vi "initialise.vi"(8 "error in (no error)":errorcluster, 11 "GenericTrajectory in":refnum<class "TrajectoryDL110413StraightLine.lvclass">) -> (0 "error out":errorcluster, 3 "GenericTrajectory out":refnum<class "TrajectoryDL110413StraightLine.lvclass">)   [LabVIEW 2010, in "TrajectoryDL110413StraightLine.lvclass"]
uses:
  TrajectoryDL110413StraightLine.lvclass
  TrajectoryDL091126GenericVoxel/TrajectoryDL091126GenericVoxel/TrajectoryDL091126GenericVoxel.lvclass
  common/enumerations/x_y_z_enumeration.ctl
  common/enumerations/functional_global_action_enum.ctl
  TrajectoryDL110413StraightLine.lvclass/TrajectoryDL110413StraightLine.ctl
  common/classes/ImageCollection/ImageCollection/ImageCollection.lvclass
  common/classes/Image/Image/Image.lvclass
  <vilib>/Analysis/1siggen.llb/Ramp Pattern by Samples.vi
  <vilib>/Analysis/NI_AALBase.lvlib
  common/classes/SpaceVector/SpaceVector/SpaceVector.lvclass
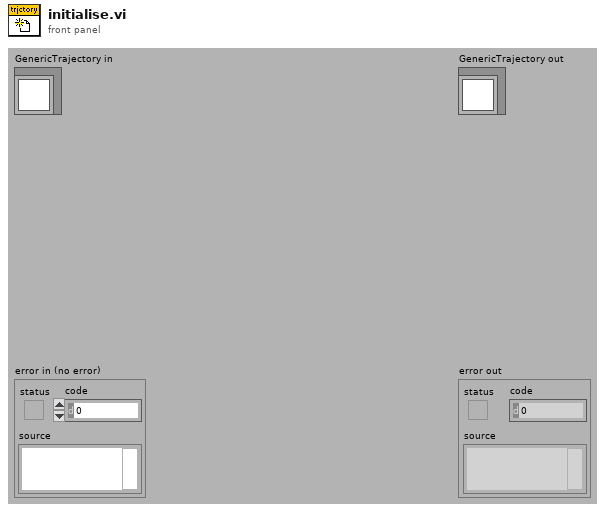
[diagram p1: front panel]
types:
  T1 = typedef "x_y_z_enumeration.ctl" = enum16{"x", "y", "z"}
  T2 = typedef "functional_global_action_enum.ctl" = enum16{"get", "set", "reset"}
  T3 = cluster{"guide points[0]":refnum<class "SpaceVector.lvclass">, "guide points[1]":refnum<class "SpaceVector.lvclass">}
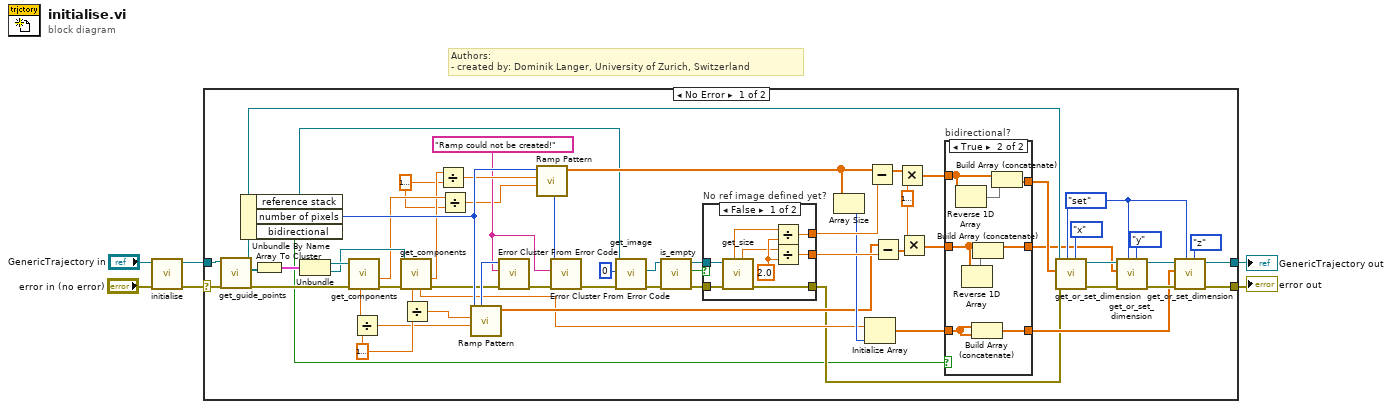
[diagram p0: block diagram]
diagram:
  # "Authors: \n- created by: Dominik Langer, University of Zurich, Switzerland"
  n1 = call-parent "initialise.vi"("error in (no error)"="error in (no error)", "GenericTrajectory in"="GenericTrajectory in") -> ("error out"=w4:errorcluster, "GenericTrajectory out"=w3:refnum<class "TrajectoryDL110413StraightLine.lvclass">)  [unwired: 8 in]
  n2 = case shown="No Error" w4 {
    selector: w4 -> [w47 w87]
    tunnel: w3 -> [w46 w88]
    tunnel: [w60 w88] -> w2
    tunnel: [w58 w87] -> w1
    frame No Error {
      w25 = dbl[unit] 1e-06 ("y")
      w19 = "Ramp could not be created!" ("error message (\"\")")
      w15 = dbl[unit] 1e-06 ("y")
      w28 = dbl[unit] 1e-06 ("y")
      w57 = functional_global_action_enum."set" ("action")
      n3 = call-dynamic "get_guide_points.vi"("error in (no error)"=w47, "TrajectoryDL110413StraightLine in"=w46) -> ("error out"=w33:errorcluster, "guide points"=w44:refnum<class "SpaceVector.lvclass">[], "TrajectoryDL110413StraightLine out"=w45:refnum<class "TrajectoryDL110413StraightLine.lvclass">)  [unwired: 7 in]
      n4 = Unbundle By Name(w45) -> ("reference stack"=w18:refnum<class "ImageCollection.lvclass">, "number of pixels"=w66:i32, "bidirectional"=w7:bool)
      n5 = Array To Cluster(array=w44) -> (cluster=w43:T3)
      n6 = Unbundle(w43) -> ("guide points[0]"=w35:refnum<class "SpaceVector.lvclass">, "guide points[1]"=w34:refnum<class "SpaceVector.lvclass">)
      n7 = call "get_components.vi"("error in (no error)"=w33, "SpaceVector in"=w35) -> ("error out"=w30:errorcluster, "x"=w27:dbl[unit], "y"=w31:dbl[unit])  [unwired: 4 in, 3 out]
      n8 = Divide(x=w31, y=w28) -> (x/y=w23:dbl)
      n9 = call "get_components.vi"("error in (no error)"=w30, "SpaceVector in"=w34) -> ("error out"=w21:errorcluster, "x"=w26:dbl[unit], "z"=w32:dbl[unit], "y"=w29:dbl[unit])  [unwired: 4 in, 2 out]
      n10 = Divide(x=w29, y=w28) -> (x/y=w22:dbl)
      n11 = Divide(x=w26, y=w25) -> (x/y=w24:dbl)
      n12 = Divide(x=w27, y=w25) -> (x/y=w17:dbl)
      n13 = call-poly <vilib>:"Ramp Pattern.vi"("start"=w23, "end"=w22, "samples"=w66) -> ("error"=w42:i32, "Ramp Pattern"=w36:dbl[])  [unwired: 7 in]
      n14 = call <vilib>:"Error Cluster From Error Code.vi"("error in (no error)"=w21, "error message (\"\")"=w19, "error code (0)"=w42) -> ("error out"=w40:errorcluster)  [unwired: 6 in]
      n15 = call-poly <vilib>:"Ramp Pattern.vi"("start"=w17, "end"=w24, "samples"=w66) -> ("error"=w41:i32, "Ramp Pattern"=w38:dbl[])  [unwired: 7 in]
      n16 = call <vilib>:"Error Cluster From Error Code.vi"("error in (no error)"=w40, "error message (\"\")"=w19, "error code (0)"=w41) -> ("error out"=w20:errorcluster)  [unwired: 6 in]
      n17 = call-dynamic "get_image.vi"("error in (no error)"=w20, "index"=0, "ImageCollection in"=w18) -> ("error out"=w52:errorcluster, "Image.lvclass"=w50:refnum<class "Image.lvclass">)  [unwired: 6 in, 1 out]
      n18 = call-dynamic "is_empty.vi"("error in (no error)"=w52, "Image in"=w50) -> ("error out"=w51:errorcluster, "emtpy?"=w48:bool, "Image out"=w49:refnum<class "Image.lvclass">)  [unwired: 7 in]
      n19 = case "No ref image defined yet?" shown="False" w48 {
        tunnel: [w85 w86] -> w8
        tunnel: [w82 _] -> w54
        tunnel: [w80 _] -> w53
        tunnel: w51 -> [w79 w86]
        tunnel: w49 -> [w78 _]
        frame False {
          w84 = 2.0 ("y")
          n20 = call-dynamic "get_size.vi"("error in (no error)"=w79, "Image in"=w78) -> ("error out"=w85:errorcluster, "physical size y"=w81:dbl, "physical size x"=w83:dbl)  [unwired: 2 in, 5 out]
          n21 = Divide(x=w83, y=w84) -> (x/y=w82:dbl)
          n22 = Divide(x=w81, y=w84) -> (x/y=w80:dbl)
        }
        frame True {
        }
      }
      n23 = Array Size(array=w38) -> (size(s)=w39:i32)
      n24 = Initialize Array(w32, w39) -> (w12:dbl[unit][])
      n25 = Subtract(x=w38, y=w54) -> (x-y=w37:dbl[])
      n26 = Subtract(x=w36, y=w53) -> (x-y=w16:dbl[])
      n27 = Multiply(x=w37, y=w15) -> (x*y=w14:dbl[unit][])
      n28 = Multiply(x=w15, y=w16) -> (x*y=w9:dbl[unit][])
      n29 = case "bidirectional?" shown="True" w7 {
        tunnel: w14 -> [w68 w77]
        tunnel: [w68 w75] -> w13
        tunnel: [w69 w73] -> w10
        tunnel: w9 -> [w69 w72]
        tunnel: w12 -> [w67 w71]
        tunnel: [w67 w70] -> w11
        frame False {
        }
        frame True {
          n30 = Reverse 1D Array(array=w77) -> (reversed array=w76:dbl[unit][])
          n31 = Reverse 1D Array(array=w72) -> (reversed array=w74:dbl[unit][])
          n32 = Build Array (concatenate)(w71, w71) -> (w70:dbl[unit][])
          n33 = Build Array (concatenate)(w72, w74) -> (w73:dbl[unit][])
          n34 = Build Array (concatenate)(w77, w76) -> (w75:dbl[unit][])
        }
      }
      n35 = call-dynamic "get_or_set_dimension.vi"("dimension"=x_y_z_enumeration."x", "action"=w57, "error in (no error)"=w8, "pixel values in (single dimension)"=w13, "GenericTrajectory in"=w45) -> ("error out"=w65:errorcluster, "GenericTrajectory out"=w64:refnum<class "TrajectoryDL110413StraightLine.lvclass">)  [unwired: 4 in, 1 out]
      n36 = call-dynamic "get_or_set_dimension.vi"("dimension"=x_y_z_enumeration."y", "action"=w57, "error in (no error)"=w65, "pixel values in (single dimension)"=w10, "GenericTrajectory in"=w64) -> ("error out"=w59:errorcluster, "GenericTrajectory out"=w61:refnum<class "TrajectoryDL110413StraightLine.lvclass">)  [unwired: 4 in, 1 out]
      n37 = call-dynamic "get_or_set_dimension.vi"("dimension"=x_y_z_enumeration."z", "action"=w57, "error in (no error)"=w59, "pixel values in (single dimension)"=w11, "GenericTrajectory in"=w61) -> ("error out"=w58:errorcluster, "GenericTrajectory out"=w60:refnum<class "TrajectoryDL110413StraightLine.lvclass">)  [unwired: 4 in, 1 out]
    }
    frame Error {
    }
  }
  "error out" <- w1
  "GenericTrajectory out" <- w2
